vi "Close.vi"(8 "error in (no error)":errorcluster caption="错误输入（无错误）", 11 "TH6402 输入":refnum<class "TH6402.lvclass">) -> (0 "error out":errorcluster caption="错误输出", 3 "TH6402 输出":refnum<class "TH6402.lvclass">)   [LabVIEW 2020, in "DP.lvlib" / "TH6402.lvclass"]
uses:
  TH6402.lvclass
  TH6402.lvclass/TH6402.ctl
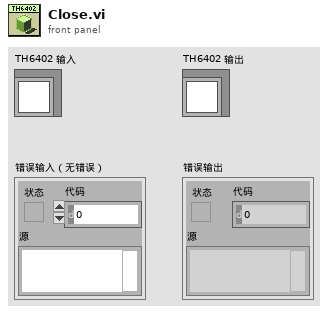
[diagram p1: front panel]
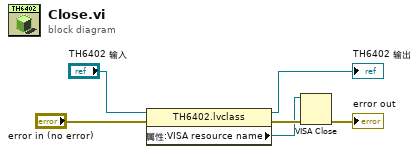
[diagram p0: block diagram]
diagram:
  n1 = property class="TH6402.lvclass"(reference="TH6402 输入", error in="error in (no error)") -> (reference out=→"TH6402 输出":refnum<class "TH6402.lvclass">, error out=w5:errorcluster, "属性:VISA resource name"=w1:refnum<visa-resource-name>)
  n2 = VISA Close(VISA resource name=w1, error in (no error)=w5) -> (error out=→"error out":errorcluster)
